vi "Chroma1A.vi"() -> ()   [LabVIEW 2015]
uses:
  <vilib>/Utility/file.llb/Write To Spreadsheet File (string).vi
panel:
  in  "Type (P_REAL)":i32(ring) items=["P_ENERGY"=4, "P_FACTOR"=3, "P_REACTIVE"=2, "P_APPARENT"=1, "P_REAL"=0]
  in  "Type (I_RMS)":i32(ring) items=["I_THD"=5, "I_CRESTFACTOR"=4, "I_INRUSH"=3, "I_PEAK-"=2, "I_PEAK+"=1, "I_RMS"=0]
  in  "Type (V_RMS)":i32(ring) items=["V_THD"=3, "V_PEAK-"=2, "V_PEAK+"=1, "V_RMS"=0]
  in  "Port Name":refnum<k15> caption="resource name"
  out "Current Data Point Count":i32
  in  "STOP":bool
  out "Graph":dbl[][](graph)
  in  "Minutes per test":dbl
  in  "Name of File":string
  in  "HOW MANY TEST":i32
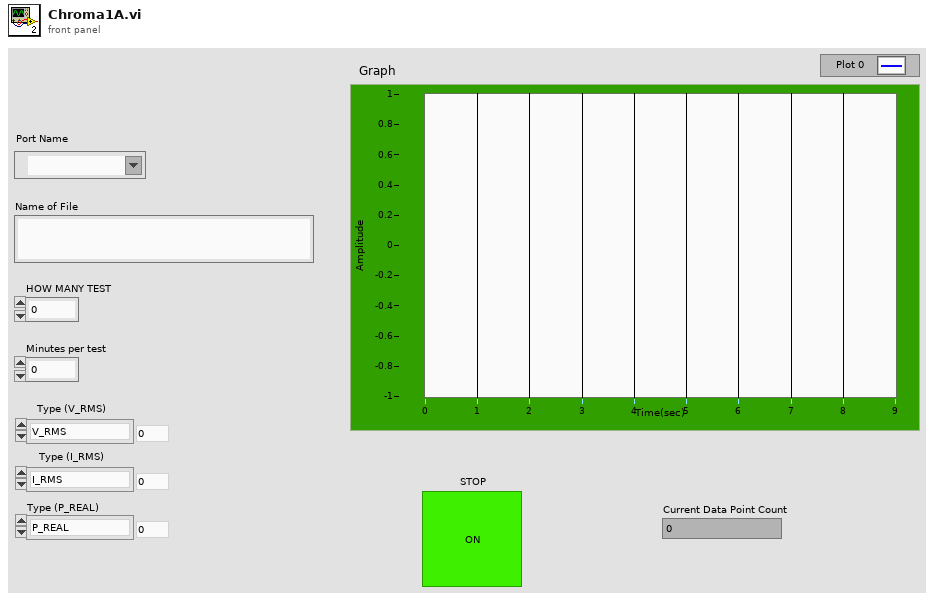
[diagram p1: front panel]
types:
  T1 = enum16{"open", "replace", "create", "open or create", "replace or create", "replace or create with confirmation"}
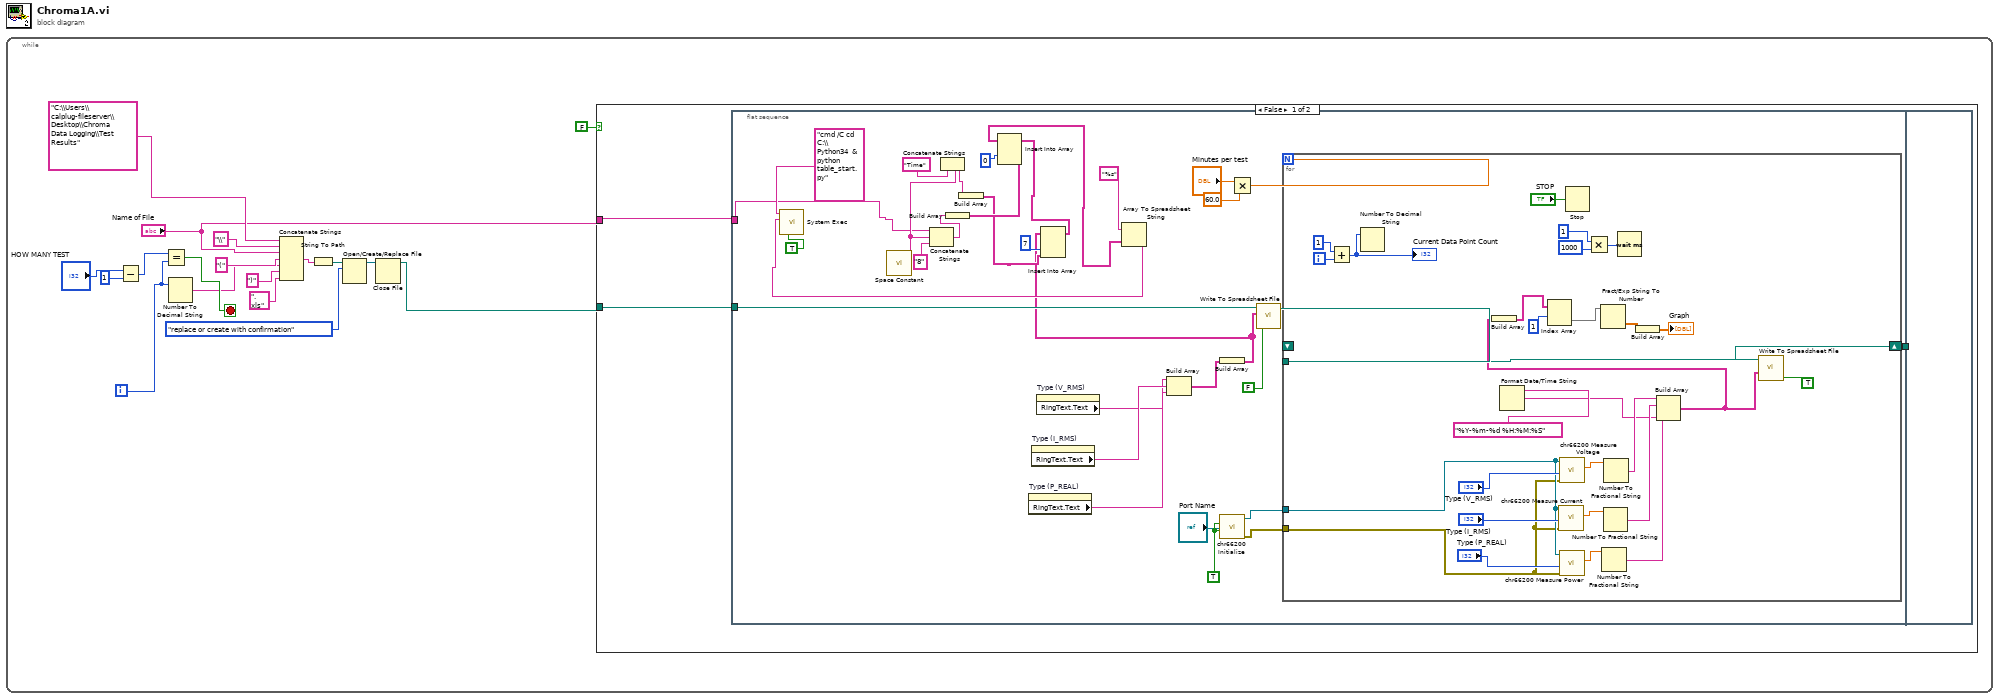
[diagram p0: block diagram]
diagram:
  n1 = while {
    i -> [w11]
    stop <- w12 stop-if-true
    n2 = Subtract(x="HOW MANY TEST", y=1) -> (x-y=w8:i32)
    n3 = Equal?(x=w8, y=w11) -> (x = y?=w12:bool)
    n4 = Number To Decimal String(number=w11) -> (decimal integer string=w3:string)  [unwired: 1 in]
    n5 = Concatenate Strings("C:\\Users\\calplug-fileserver\\Desktop\\Chroma Data Logging\\Test Results" ("string"), "\\" ("string"), "Name of File", "(" ("string"), w3, ")" ("string"), ".xls" ("string")) -> (w15:string)
    n6 = String To Path(string=w15) -> (path=w16:path)
    n7 = Open/Create/Replace File(file path (use dialog)=w16, operation (0:open)=T1."replace or create with confirmation") -> (refnum out=w14:refnum<file>)  [unwired: 4 in, 2 out]
    n8 = Close File(refnum=w14) -> (path=w13:path)  [unwired: 1 in, 1 out]
    n9 = case shown="False" FALSE {
      tunnel: w13 -> [w21 _]
      tunnel: "Name of File" -> [w19 _]
      frame False {
        n10 = flat-sequence {
          tunnel: w21 -> [w52]
          tunnel: [w53] -> w20
          tunnel: w19 -> [w34]
          tunnel: w20 -> [_]
          frame #0 {
            w24 = TRUE
            n11 = call <vilib>:"Space Constant.vi"() -> ("String"=w39:string)
            n12 = Concatenate Strings(w34, w39, "8") -> (w41:string)
            n13 = Concatenate Strings("Time", w39) -> (w36:string)
            n14 = Build Array(w41) -> (w42:string[])
            n15 = Build Array(w36) -> (w37:string[])
            n16 = property on="Type (P_REAL)" class="Ring (strict)"() -> ("RingText.Text"=w30:string)  [unwired: 2 in, 2 out]
            n17 = property on="Type (I_RMS)" class="Ring (strict)"() -> ("RingText.Text"=w31:string)  [unwired: 2 in, 2 out]
            n18 = property on="Type (V_RMS)" class="Ring (strict)"() -> ("RingText.Text"=w27:string)  [unwired: 2 in, 2 out]
            n19 = Build Array(w27, w31, w30) -> (w29:string[])
            n20 = Build Array(w29) -> (w28:string[][])
            n21 = Insert Into Array(array=w28, index (col)=7, new element=w37) -> (w44:string[][])  [unwired: 1 in]
            n22 = Insert Into Array(array=w44, index (col)=0, new element=w42) -> (w32:string[][])  [unwired: 1 in]
            n23 = Array To Spreadsheet String(array=w32, 3:"%s") -> (spreadsheet string=w33:string)  [unwired: 1 in]
            n24 = call <vilib>:"System Exec.vi"("run minimized? (F)"=TRUE, "standard input"=w33, "command line"="cmd /C cd C:\\Python34  & python table_start.py") -> ()  [unwired: 5 in, 4 out]
            n25 = call <instrlib>:"chr66200 Initialize.vi"("Reset Device (Yes)"=w24, "ID Query (Yes)"=w24, "resource name"="Port Name") -> ("error out"=w22:errorcluster, "instrument handle out"=w23:refnum<k15>)  [unwired: 7 in]
            n26 = Multiply(x="Minutes per test", y=60.0) -> (x*y=w50:dbl)
            n27 = call-poly <vilib>:"Write To Spreadsheet File.vi"("append to file? (new file:F)"=FALSE, "2D data"=w28, "file path (dialog if empty)"=w52) -> ("new file path (Not A Path if cancelled)"=w51:path)  [unwired: 5 in]
            n28 = for {
              N: w50 -> [_]
              tunnel: w51 -> [w77]
              shift-right: [w75] -> w53
              shift-left: _ -> [_]
              tunnel: w23 -> [w55]
              tunnel: w22 -> [w54]
              i -> [w79]
              n29 = Add(x=1, y=w79) -> (x+y=w80:i32)
              "Current Data Point Count" <- w80
              n30 = Number To Decimal String(number=w80) -> ()  [unwired: 1 in, 1 out]
              n31 = Format Date/Time String(time format string (%c)="%Y-%m-%d %H:%M:%S") -> (date/time string=w57:string)  [unwired: 2 in]
              n32 = call <instrlib>:"chr66200 Measure Current.vi"("error in (no error)"=w54, "Type (I_RMS)"="Type (I_RMS)", "instrument handle"=w55) -> ("Read Value"=w62:dbl)  [unwired: 6 in, 2 out]
              n33 = call <instrlib>:"chr66200 Measure Voltage.vi"("error in (no error)"=w54, "Type (V_RMS)"="Type (V_RMS)", "instrument handle"=w55) -> ("Read Value"=w63:dbl)  [unwired: 6 in, 2 out]
              n34 = call <instrlib>:"chr66200 Measure Power.vi"("error in (no error)"=w54, "Type (P_REAL)"="Type (P_REAL)", "instrument handle"=w55) -> ("Read Value"=w61:dbl)  [unwired: 6 in, 2 out]
              n35 = Stop(stop? (T)="STOP") -> ()
              n36 = Multiply(x=u32 1 ("Interval of Data Collection (sec)"), y=u32 1000) -> (x*y=w81:u32)
              n37 = Number To Fractional String(number=w61) -> (F-format string=w58:string)  [unwired: 3 in]
              n38 = Number To Fractional String(number=w62) -> (F-format string=w59:string)  [unwired: 3 in]
              n39 = Number To Fractional String(number=w63) -> (F-format string=w60:string)  [unwired: 3 in]
              n40 = Wait (ms)(milliseconds to wait=w81) -> ()  [unwired: 1 out]
              n41 = Build Array(w60, w59, w58, w57) -> (w56:string[])
              n42 = Build Array(w56) -> (w67:string[][])
              n43 = Index Array(array=w67, index (row)=1) -> (element=w68:string[])  [unwired: 1 in]
              n44 = Fract/Exp String To Number(string=w68) -> (number=w70:dbl[])  [unwired: 3 in, 1 out]
              n45 = Build Array(w70) -> (→"Graph":dbl[][])
              n46 = call-poly <vilib>:"Write To Spreadsheet File.vi"("append to file? (new file:F)"=TRUE, "1D data"=w56, "file path (dialog if empty)"=w77) -> ("new file path (Not A Path if cancelled)"=w75:path)  [unwired: 5 in]
            }
          }
          frame #1 {
          }
        }
      }
      frame True {
      }
    }
  }
